vi "FileIO-Save Dialog.vi"(6 "Overwrite prompt?":bool=TRUE, 7 "Default Folder":path, 8 "error in":errorcluster, 10 "pattern (all files)":string="*.ini", 11 "Start path":path) -> (0 "error out":errorcluster, 1 "cancelled":bool, 3 "selected path":path)   [LabVIEW 2020]
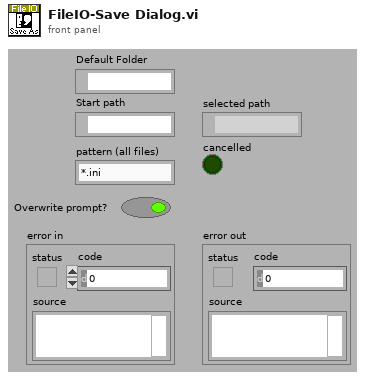
[diagram p1: front panel]
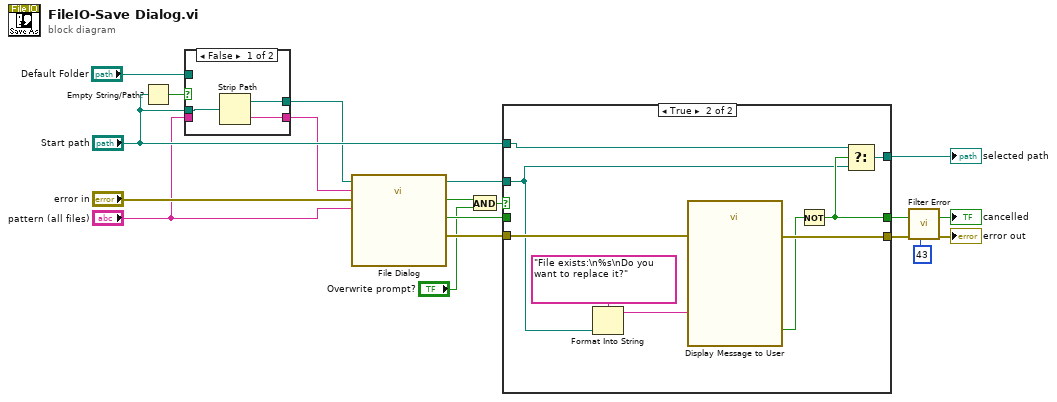
[diagram p0: block diagram]
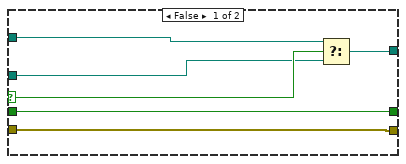
[diagram p3: hidden frame]
diagram:
  n1 = Empty String/Path?(string/path="Start path") -> (empty?=w6:bool)
  n2 = case shown="False" w6 {
    tunnel: "Default Folder" -> [_ w23]
    tunnel: "Start path" -> [w21 _]
    tunnel: [w20 w23] -> w3
    tunnel: [w19 w22] -> w2
    tunnel: "pattern (all files)" -> [_ w22]
    frame False {
      n3 = Strip Path(path=w21) -> (stripped path=w20:path, name=w19:string)
    }
    frame True {
    }
  }
  n4 = call "File Dialog"("start path"=w3, "default name"=w2, "error in"="error in", "pattern (all files)"="pattern (all files)") -> ("selected path"=w13:path, "exists"=w17:bool, "cancelled"=w12:bool, "error out"=w14:errorcluster)  [unwired: 8 in]
  n5 = And(x=w17, y="Overwrite prompt?") -> (x .and. y?=w8:bool)
  n6 = case shown="True" w8 {
    selector: w8 -> [w26 _]
    tunnel: w14 -> [w28 w38]
    tunnel: w13 -> [w24 w30]
    tunnel: [w29 w32] -> w11
    tunnel: w12 -> [w29 _]
    tunnel: [w28 w35] -> w10
    tunnel: "Start path" -> [w25 w31]
    tunnel: [w27 w34] -> w9
    frame False {
      n7 = Select(t=w25, s=w26, f=w24) -> (s? t:f=w27:path)
    }
    frame True {
      n8 = Format Into String(format string="File exists:\n%s\nDo you want to replace it?", w30) -> (resulting string=w36:string)  [unwired: 2 in, 1 out]
      n9 = call "Display Message to User"("error in (no error)"=w38, "Message"=w36) -> ("error out"=w35:errorcluster, "Yes"=w33:bool)  [unwired: 8 in]
      n10 = Not(x=w33) -> (.not. x?=w32:bool)
      n11 = Select(t=w31, s=w32, f=w30) -> (s? t:f=w34:path)
    }
  }
  "selected path" <- w9
  "cancelled" <- w11
  n12 = call "Filter Error.vi"("error in (no error)"=w10, "code to ignore"=43) -> ("error out"=→"error out":errorcluster)  [unwired: 9 in]
